vi "Get Named Unbundlers.vi"(7 "Owner (Default - Block Diagram)":refnum<vi>, 8 "error in (no error)":errorcluster, 11 "VI in":refnum<vi>) -> (0 "error out":errorcluster, 1 "# of Refs":i32, 2 "NamedUnbundlers":refnum<vi>[](array[refnum]), 3 "VI out":refnum<vi>)   [LabVIEW 2018, in "Scripting.lvlib"]
uses:
  Scripting.lvlib
  <vilib>/Utility/traverseref.llb/TRef TravTarget.ctl
  <vilib>/Utility/traverseref.llb/VI Scripting - Traverse.lvlib
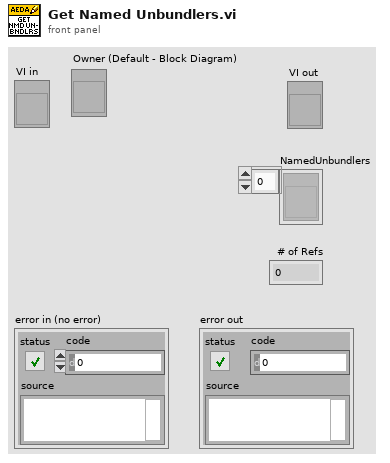
[diagram p1: front panel]
types:
  T1 = typedef "TRef TravTarget.ctl" = enum16{"FP", "BD", "Other"}
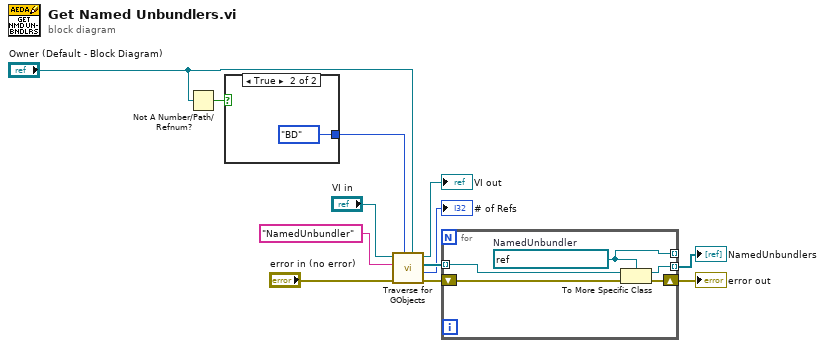
[diagram p0: block diagram]
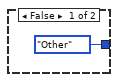
[diagram p2: hidden frame]
diagram:
  n1 = Not A Number/Path/Refnum?(number/path/refnum="Owner (Default - Block Diagram)") -> (NaN/Path/Refnum?=w5:bool)
  n2 = case shown="True" w5 {
    tunnel: [TRef_TravTarget."Other" ("Traverse Target") TRef_TravTarget."BD" ("Traverse Target")] -> w4
    frame False {
    }
    frame True {
    }
  }
  n3 = call <vilib>:"Traverse for GObjects.vi"("Other Refnum"="Owner (Default - Block Diagram)", "Traverse Target"=w4, "error in (no error)"="error in (no error)", "Class Name"="NamedUnbundler", "VI Refnum"="VI in") -> ("error out"=w10:errorcluster, "# of Refs"=→"# of Refs":i32, "References"=w8:refnum<vi>[], "dup VI Refnum"=→"VI out":refnum<vi>)  [unwired: 3 in]
  n4 = for {
    tunnel: w8 -> [w17] mode=indexing
    shift-right: [w18] -> w9
    shift-left: w10 -> [w19]
    tunnel: [w16] -> w1 mode=indexing
    tunnel: [w15] -> _ mode=indexing
    w15 = refnum<vi> refnum  # NamedUnbundler
    n5 = To More Specific Class(target class=w15, reference=w17, error in=w19) -> (specific class reference=w16:refnum<vi>, error out=w18:errorcluster)
  }
  "error out" <- w9
  "NamedUnbundlers" <- w1
